vi "insert.vi"(8 "error in":errorcluster, 11 "MG090623BinningImageAssembler in":refnum<class "ImageAssemblerMG090623Binning.lvclass">) -> (0 "error out":errorcluster, 3 "MG090623BinningImageAssembler out":refnum<class "ImageAssemblerMG090623Binning.lvclass">)   [LabVIEW 2010, in "ImageAssemblerMG090623Binning.lvclass"]
uses:
  ImageAssemblerMG090623Binning.lvclass
  common/classes/Image/Image/Image.lvclass
  ImageAssemblerMG090623Binning.lvclass/ImageAssemblerMG090623Binning.ctl
  common/classes/ErrorController/ErrorController/class_data.vi
  ImageAssemblerDL090211Scaffold/ImageAssemblerDL090211Scaffold/ImageAssemblerDL090211Scaffold.lvclass
  common/classes/ErrorController/ErrorController/ErrorController.lvclass
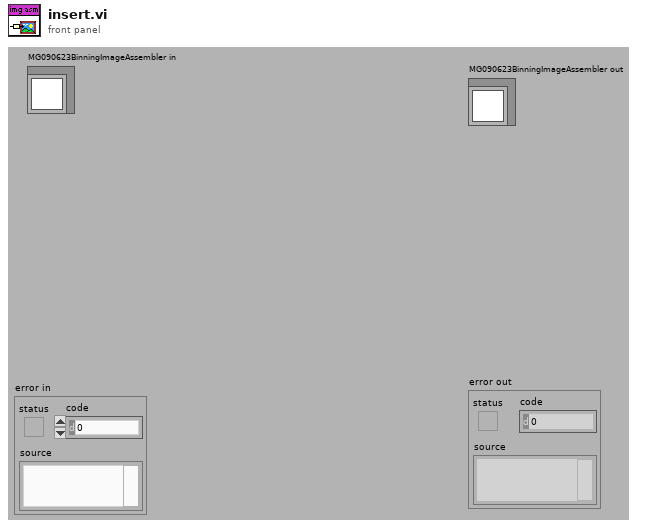
[diagram p1: front panel]
types:
  T1 = typedef "Image Type" = u32
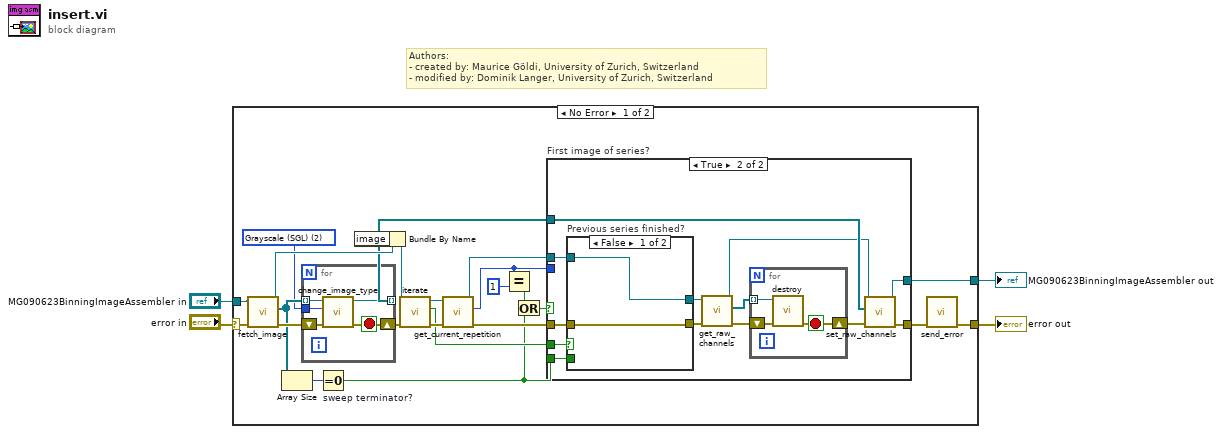
[diagram p0: block diagram]
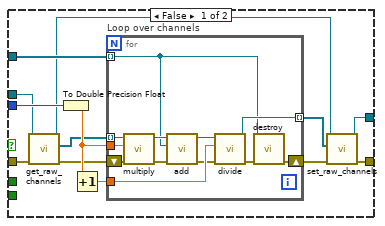
[diagram p2: hidden frame]
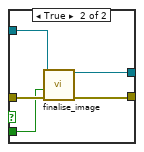
[diagram p3: hidden frame]
diagram:
  # "Authors: \n- created by: Maurice Göldi, University of Zurich, Switzerland\n- modified by: Dominik Langer, University of Zurich, Switzerland"
  n1 = case shown="No Error" "error in" {
    selector: "error in" -> [w23 w82]
    tunnel: [w6 w82] -> w3
    tunnel: [w27 w81] -> w4
    tunnel: "MG090623BinningImageAssembler in" -> [w22 w81]
    frame No Error {
      w7 = T1 2 items=["Grayscale (U8)", "Grayscale (I16)", "Grayscale (SGL)", "Complex (CSG)", "RGB (U32)", "HSL (U32)", "RGB (U64)", "Grayscale (U16)"] ("target image type")
      n2 = call-dynamic "fetch_image.vi"("error in (no error)"=w23, "GenericToplevelComponent in"=w22) -> ("error out"=w11:errorcluster, "image (channels)"=w9:refnum<class "Image.lvclass">[], "GenericToplevelComponent out"=w25:refnum<class "ImageAssemblerMG090623Binning.lvclass">)  [unwired: 4 in, 3 out]
      n3 = Array Size(array=w9) -> (size(s)=w26:i32)
      n4 = for {
        tunnel: w9 -> [w31] mode=indexing
        shift-right: [w28] -> w10
        shift-left: w11 -> [w32]
        tunnel: [w30] -> w8 mode=indexing
        tunnel: w7 -> [w29]
        stop <- w28 stop-if-true
        n5 = call "change_image_type.vi"("error in (no error)"=w32, "target image type"=w29, "Image in"=w31) -> ("error out"=w28:errorcluster, "Image out"=w30:refnum<class "Image.lvclass">)  [unwired: 7 in]
      }
      n6 = Equal To 0? "sweep terminator?"(x=w26) -> (x = 0?=w12:bool)
      n7 = Bundle By Name(cluster=w25, "image"=w8) -> (w24:refnum<class "ImageAssemblerMG090623Binning.lvclass">)
      n8 = call-dynamic "iterate.vi"("error in (no error)"=w10, "MG090623BinningImageAssembler in"=w24) -> ("error out"=w21:errorcluster, "finished?"=w17:bool, "MG090623BinningImageAssembler out"=w19:refnum<class "ImageAssemblerMG090623Binning.lvclass">)  [unwired: 7 out]
      n9 = call "get_current_repetition.vi"("error in (no error)"=w21, "DL090211ImageAssemblerScaffold.lvclass in"=w19) -> ("error out"=w20:errorcluster, "current repetition"=w16:i32, "DL090211ImageAssemblerScaffold.lvclass out"=w18:refnum<class "ImageAssemblerMG090623Binning.lvclass">)  [unwired: 7 in]
      n10 = Equal?(x=w16, y=1) -> (x = y?=w14:bool)
      n11 = Or(x=w14, y=w12) -> (x .or. y?=w13:bool)
      n12 = case "First image of series?" shown="True" w13 {
        tunnel: w20 -> [w34 w70]
        tunnel: [w44 w69] -> w5
        tunnel: w8 -> [w45 w63]
        tunnel: w18 -> [w36 w66]
        tunnel: [w43 w68] -> w27
        tunnel: w17 -> [_ w67]
        tunnel: w16 -> [w42 _]
        tunnel: w12 -> [_ w64]
        frame False {
          n13 = call-dynamic "get_raw_channels.vi"("error in (no error)"=w34, "DL090211ImageAssemblerScaffold.lvclass in"=w36) -> ("error out"=w33:errorcluster, "raw channels"=w37:refnum<class "Image.lvclass">[], "DL090211ImageAssemblerScaffold.lvclass out"=w35:refnum<class "ImageAssemblerMG090623Binning.lvclass">)  [unwired: 7 out]
          n14 = To Double Precision Float(number=w42) -> (double precision float=w39:dbl)
          n15 = Increment(x=w39) -> (x+1=w38:dbl)
          n16 = for "Loop over channels" {
            tunnel: w37 -> [w56] mode=indexing
            tunnel: [w54] -> w40 mode=indexing
            shift-right: [w47] -> w41
            shift-left: w33 -> [w57]
            tunnel: w45 -> [w46] mode=indexing
            tunnel: w39 -> [w53]
            tunnel: w38 -> [w52]
            n17 = call-dynamic "multiply.vi"("error in (no error)"=w57, "factor"=w53, "Image in"=w56) -> ("error out"=w51:errorcluster, "Image out"=w50:refnum<class "Image.lvclass">)  [unwired: 1 in, 6 out]
            n18 = call-dynamic "add.vi"("error in (no error)"=w51, "addend"=w46, "Image in"=w50) -> ("error out"=w49:errorcluster, "Image out"=w55:refnum<class "Image.lvclass">)  [unwired: 1 in, 6 out]
            n19 = call-dynamic "divide.vi"("error in (no error)"=w49, "divisor"=w52, "Image in"=w55) -> ("error out"=w48:errorcluster, "Image out"=w54:refnum<class "Image.lvclass">)  [unwired: 1 in, 6 out]
            n20 = call-dynamic "destroy.vi"("error in (no error)"=w48, "Image in"=w46) -> ("error out"=w47:errorcluster)  [unwired: 8 in, 1 out]
          }
          n21 = call "set_raw_channels.vi"("error in (no error)"=w41, "raw channels"=w40, "DL090211ImageAssemblerScaffold.lvclass in"=w35) -> ("error out"=w44:errorcluster, "DL090211ImageAssemblerScaffold.lvclass out"=w43:refnum<class "ImageAssemblerMG090623Binning.lvclass">)  [unwired: 7 in]
        }
        frame True {
          n22 = case "Previous series finished?" shown="False" w67 {
            tunnel: w70 -> [w74 w80]
            tunnel: [w74 w77] -> w62
            tunnel: [w75 w78] -> w60
            tunnel: w66 -> [w75 w79]
            tunnel: w64 -> [_ w76]
            frame False {
            }
            frame True {
              n23 = call-dynamic "finalise_image.vi"("error in (no error)"=w80, "end of sweep?"=w76, "ImageAssemblerMG090623Binning in"=w79) -> ("error out"=w77:errorcluster, "ImageAssemblerMG090623Binning out"=w78:refnum<class "ImageAssemblerMG090623Binning.lvclass">)  [unwired: 7 in]
            }
          }
          n24 = call-dynamic "get_raw_channels.vi"("error in (no error)"=w62, "DL090211ImageAssemblerScaffold.lvclass in"=w60) -> ("error out"=w61:errorcluster, "raw channels"=w58:refnum<class "Image.lvclass">[], "DL090211ImageAssemblerScaffold.lvclass out"=w59:refnum<class "ImageAssemblerMG090623Binning.lvclass">)  [unwired: 7 out]
          n25 = for {
            shift-right: [w71] -> w65
            shift-left: w61 -> [w73]
            tunnel: w58 -> [w72] mode=indexing
            stop <- w71 stop-if-true
            n26 = call-dynamic "destroy.vi"("error in (no error)"=w73, "Image in"=w72) -> ("error out"=w71:errorcluster)  [unwired: 8 in, 1 out]
          }
          n27 = call "set_raw_channels.vi"("error in (no error)"=w65, "raw channels"=w63, "DL090211ImageAssemblerScaffold.lvclass in"=w59) -> ("error out"=w69:errorcluster, "DL090211ImageAssemblerScaffold.lvclass out"=w68:refnum<class "ImageAssemblerMG090623Binning.lvclass">)  [unwired: 7 in]
        }
      }
      n28 = call "send_error.vi"("error in (no error)"=w5) -> ("error out"=w6:errorcluster)  [unwired: 10 in]
    }
    frame Error {
    }
  }
  "error out" <- w3
  "MG090623BinningImageAssembler out" <- w4
